vi "Read Humidifiers.vi"(8 "error in (no error)":errorcluster, 11 "cCRDS in":refnum<class "cCRDS.lvclass">) -> (0 "error out":errorcluster, 2 "Humidifiers":T1, 3 "cCRDS out":refnum<class "cCRDS.lvclass">)   [LabVIEW 2012, in "cCRDS.lvclass"]
uses:
  cCRDS.lvclass
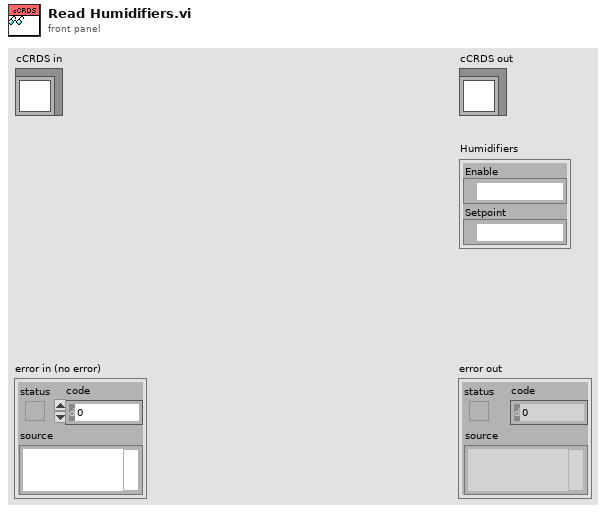
[diagram p1: front panel]
types:
  T1 = cluster{"Enable":refnum<k21>, "Setpoint":refnum<k21>}
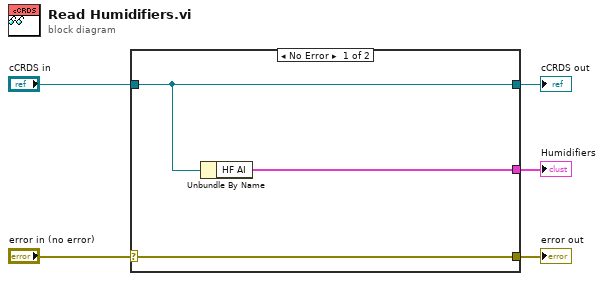
[diagram p0: block diagram]
diagram:
  n1 = case shown="No Error" "error in (no error)" {
    selector: "error in (no error)" -> [w8 w9]
    tunnel: [w8 w9] -> w4
    tunnel: [w7 w10] -> w2
    tunnel: "cCRDS in" -> [w7 w10]
    tunnel: [w6 _] -> w1
    frame No Error {
      n2 = Unbundle By Name(w7) -> ("HF AI"=w6:cluster{"AI":refnum<k21>, "Gate CO":refnum<k21>})
    }
    frame Error {
    }
  }
  "error out" <- w4
  "cCRDS out" <- w2
  "Humidifiers" <- w1
